vi "Get_Parameter Json.vi"(8 "error in (no error)":errorcluster caption="entrée d'erreur (pas d'erreur)", 11 "Class Instrument DIO en entrée":refnum<class "Class Instrument Ana.lvclass">) -> (0 "error out":errorcluster caption="sortie d'erreur", 2 "Parameter Json":string, 3 "Class Instrument DIO en sortie":refnum<class "Class Instrument Ana.lvclass">)   [LabVIEW 2020, in "Library Instrument & Equipement.lvlib" / "Library Instruments.lvlib" / "Class Instrument Ana.lvclass"]
uses:
  Class Instrument Ana.lvclass
  Class Instrument Ana.lvclass/Class Instrument Ana.ctl
  JSON API/Variant JSON/Variant to JSON.vi
  JSON API/JSON Value/Get Item by name array.vi
  Instrument (Default)/Class Instrument (Default).lvclass
  JSON API/JSON Value/JSON Value.lvclass
  JSON API/Get Polymorphic/JSON GetSet.lvlib
  JSON API/Variant JSON/Variant JSON.lvlib
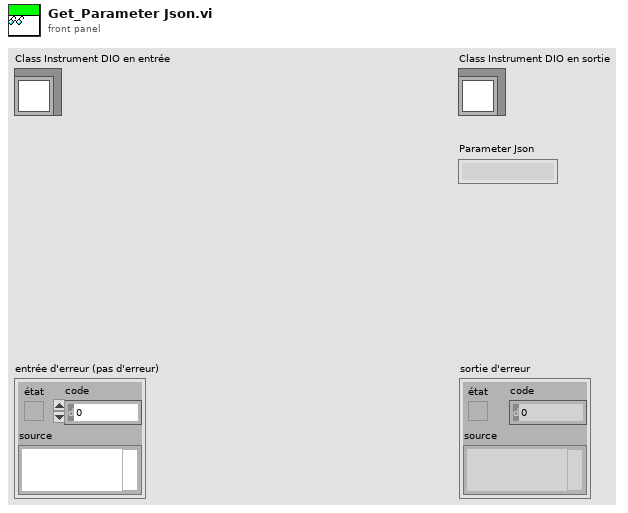
[diagram p1: front panel]
types:
  T1 = cluster{"Device_Com_Port":string, "Rate":u16, "Nb Sample":u16, "Voltage Max":dbl, "Voltage Min":dbl, "Input terminal Configuration":string, "Channel":u8[], "Continuous":bool, "Nb Data_To_Read":i16, "Class Ana":refnum<class "Class Ana (Default).lvclass">}
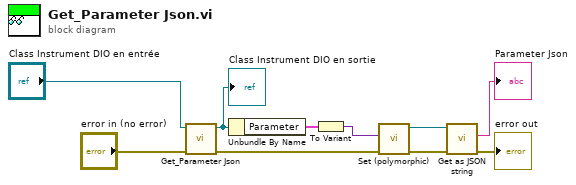
[diagram p0: block diagram]
diagram:
  n1 = call-parent "Get_Parameter Json.vi"("error in (no error)"="error in (no error)", "Class Instrument (Default) en entrée"="Class Instrument DIO en entrée") -> ("error out"=w3:errorcluster, "Class Instrument (Default) en sortie"=w4:refnum<class "Class Instrument Ana.lvclass">)  [unwired: 7 in, 1 out]
  "Class Instrument DIO en sortie" <- w4
  n2 = Unbundle By Name(w4) -> ("Parameter"=w5:T1)
  n3 = To Variant(anything=w5) -> (Variant=w8:variant)
  n4 = call-poly "Set (polymorphic).vi"("error in (no error)"=w3, "Variant"=w8) -> ("error out"=w6:errorcluster, "JSON Value out"=w7:refnum<class "JSON Value.lvclass">)  [unwired: 8 in]
  n5 = call "Get as JSON string.vi"("error in (no error)"=w6, "JSON Value in"=w7) -> ("error out"=→"error out":errorcluster, "<JSON>"=→"Parameter Json":string)  [unwired: 8 in]
